vi "getAxisObject.vi"(8 "error in (no error)":errorcluster, 10 "Axis Letter":string, 11 "Controller in":refnum<class "Controller.lvclass">) -> (0 "error out":errorcluster, 2 "Axis Object":refnum<class "Axis.lvclass">, 3 "Controller out":refnum<class "Controller.lvclass">)   [LabVIEW 2019, in "Controller.lvclass"]
uses:
  Controller.lvclass
  Axis/Axis.lvclass
  Controller.lvclass/Controller.ctl
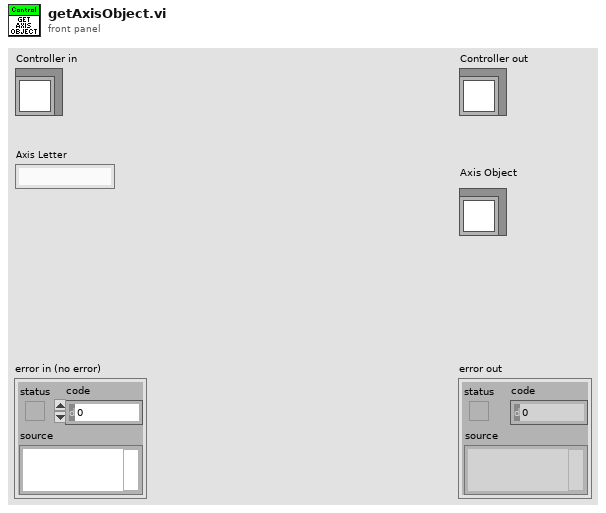
[diagram p1: front panel]
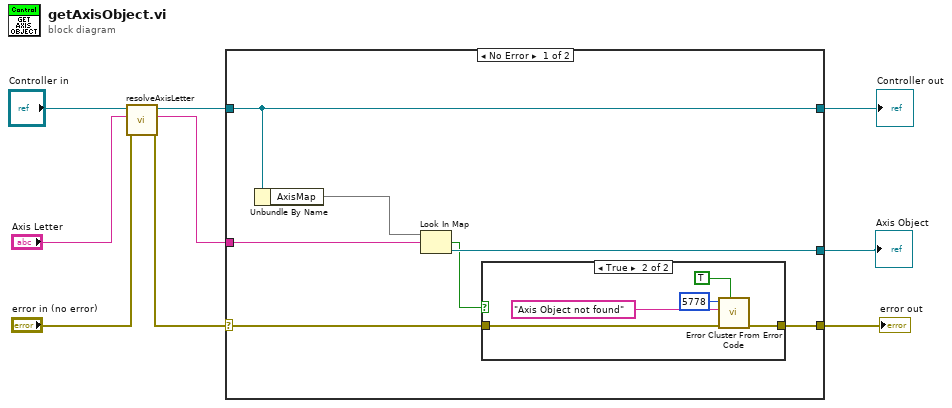
[diagram p0: block diagram]
diagram:
  n1 = call "resolveAxisLetter.vi"("error in (no error)"="error in (no error)", "Axis Letter in"="Axis Letter", "Controller in"="Controller in") -> ("error out"=w1:errorcluster, "Axis Letter out"=w5:string, "Controller out"=w3:refnum<class "Controller.lvclass">)  [unwired: 6 in]
  n2 = case shown="No Error" w1 {
    selector: w1 -> [w10 w24]
    tunnel: [w12 w24] -> w9
    tunnel: [w13 w23] -> w8
    tunnel: w3 -> [w13 w23]
    tunnel: w5 -> [w15 _]
    tunnel: [w16 _] -> w7
    frame No Error {
      n3 = Unbundle By Name(w13) -> ("AxisMap"=w14:map{string, refnum<class "Axis.lvclass">})
      n4 = Look In Map(map=w14, key=w15) -> (key not found?=w11:bool, value=w16:refnum<class "Axis.lvclass">)  [unwired: 1 in]
      n5 = case shown="True" w11 {
        tunnel: [w17 w22] -> w12
        tunnel: w10 -> [w17 w21]
        frame False {
        }
        frame True {
          n6 = call <vilib>:"Error Cluster From Error Code.vi"("show call chain? (False)"=TRUE, "error in (no error)"=w21, "error message (\"\")"="Axis Object not found" ("error message (\"\")"), "error code (0)"=5778) -> ("error out"=w22:errorcluster)  [unwired: 5 in]
        }
      }
    }
    frame Error {
    }
  }
  "error out" <- w9
  "Controller out" <- w8
  "Axis Object" <- w7
